vi "数据库更新.vi"(0 "设备号":string(combo)="01", 5 "数据":string[](array[string])=["123456", "ZHANG", "1", "1", "20150718", "20150719", "5", "Q14073-01", "100", "100", "100", "100", "200", "200", "200", "300", "300", "300", "300", "300", "300", "300", "300"], 11 "error in (no error)":errorcluster) -> (15 "error out":errorcluster)   [LabVIEW 2013]
panel:
  out "连接的字符串":string
  in  "数据名":string[](array[string])=["CZZ", "WC", "HG", "KSSJ", "JSSJ", "FGCS", "SBID", "Date1", "Date2", "Date3", "Date4", "Date5", "Date6", "Date7", "Date8", "Date9", "Date10"]
  # "CZZ\nWC\nHG\nKSSJ\nJSSJ\nFGCS\nSBID\nDate1\nDate2\nDate3\nDate4\nDate5\nDate6\nDate7\nDate8\nDate9\nDate10"
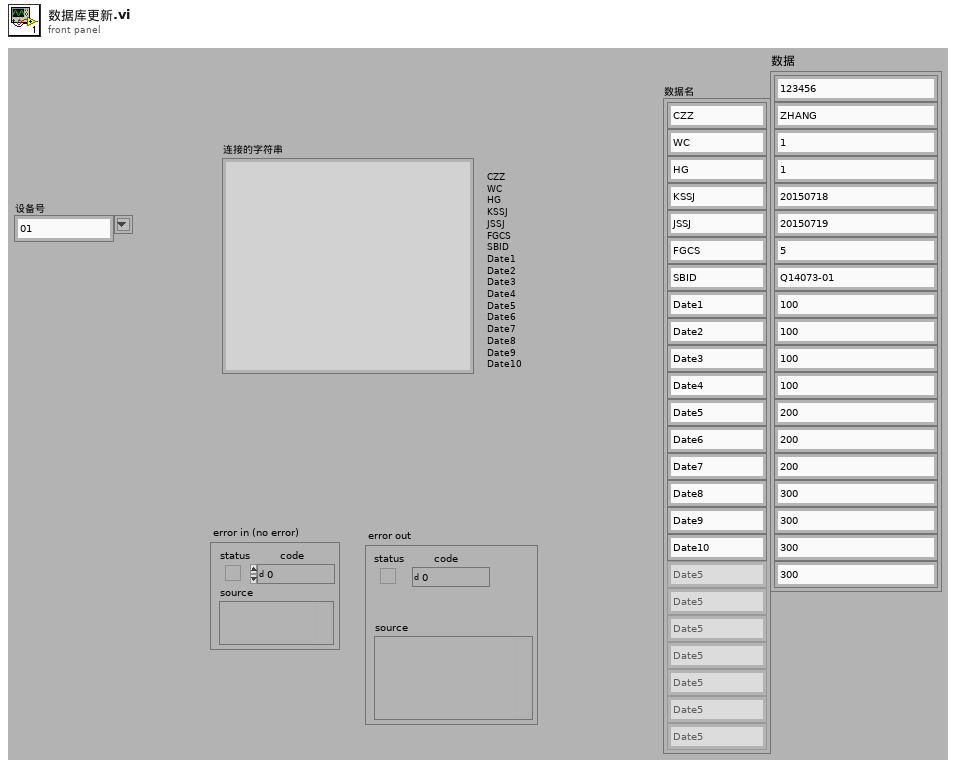
[diagram p1: front panel]
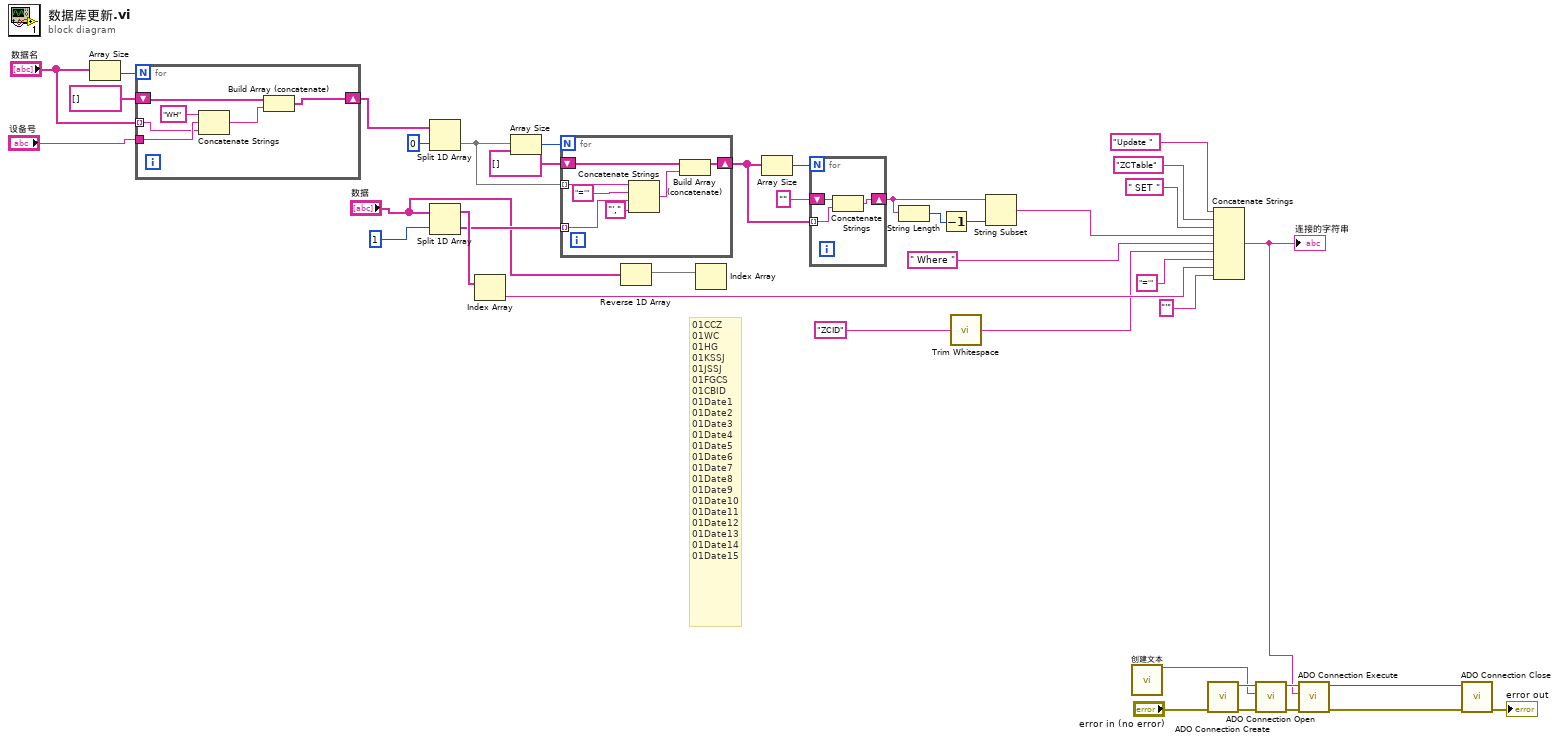
[diagram p0: block diagram]
diagram:
  # "01CCZ\n01WC\n01HG\n01KSSJ\n01JSSJ\n01FGCS\n01CBID\n01Date1\n01Date2\n01Date3\n01Date4\n01Date5\n01Date6\n01Date7\n01Date8\n01Date9\n01Date10\n01Date11\n01Date12\n01Date13\n01Date14\n01Date15"
  n1 = Array Size(array="数据名") -> (size(s)=w12:i32)
  n2 = for {
    N: w12 -> [_]
    tunnel: "数据名" -> [w42] mode=indexing
    shift-right: [w44] -> w8
    shift-left: string[] [] -> [w46]
    tunnel: "设备号" -> [w43]
    n3 = Concatenate Strings("WH" ("字符串"), w43, w42) -> (w45:string)
    n4 = Build Array (concatenate)(w46, w45) -> (w44:string[])
  }
  n5 = Split 1D Array(array=w8, index=0 ("索引")) -> (second subarray=w28:string[])  [unwired: 1 out]
  n6 = Split 1D Array(array="数据", index=1 ("索引列")) -> (first subarray=w30:string[], second subarray=w27:string[])
  n7 = Index Array(array=w30) -> (element=w15:string)  [unwired: 1 in]
  n8 = Array Size(array=w28) -> (size(s)=w29:i32)
  n9 = for {
    N: w29 -> [_]
    tunnel: w28 -> [w53] mode=indexing
    shift-right: [w50] -> w25
    shift-left: string[] [] -> [w49]
    tunnel: w27 -> [w48] mode=indexing
    n10 = Concatenate Strings(w53, "='" ("字符串"), w48, "'," ("字符串")) -> (w51:string)
    n11 = Build Array (concatenate)(w49, w51) -> (w50:string[])
  }
  n12 = Reverse 1D Array(array="数据") -> (reversed array=w7:string[])
  n13 = Index Array(array=w7) -> ()  [unwired: 1 in, 1 out]
  n14 = Array Size(array=w25) -> (size(s)=w26:i32)
  n15 = for {
    N: w26 -> [_]
    tunnel: w25 -> [w56] mode=indexing
    shift-right: [w55] -> w24
    shift-left: "" -> [w54]
    n16 = Concatenate Strings(w54, w56) -> (w55:string)
  }
  n17 = String Length(string=w24) -> (length=w5:i32)
  n18 = Decrement(x=w5) -> (x-1=w4:i32)
  n19 = call <vilib>:"Trim Whitespace.vi"("string"="ZCID" ("索引列名")) -> ("trimmed string"=w1:string)  [unwired: 1 in]
  n20 = String Subset(string=w24, length (rest)=w4) -> (substring=w3:string)  [unwired: 1 in]
  n21 = call "创建文本"() -> ("Result"=w32:string)  [unwired: 14 in, 1 out]
  n22 = call "ADO Connection Create.vi"("error in (no error)"="error in (no error)") -> ("error out"=w39:errorcluster, "ADODB._Connection Out"=w38:refnum<k7>)  [unwired: 9 out]
  n23 = Concatenate Strings("Update " ("字符串"), "ZCTable" ("数据库名"), " SET " ("字符串"), w3, " Where " ("字符串"), w1, "='" ("字符串"), w15, "'" ("字符串")) -> (w6:string)
  "连接的字符串" <- w6
  n24 = call "ADO Connection Open.vi"("error in (no error)"=w39, "ConnectionString"=w32, "ADODB._Connection In"=w38) -> ("error out"=w37:errorcluster, "ADODB._Connection Out"=w36:refnum<k7>)  [unwired: 7 out]
  n25 = call "ADO Connection Execute.vi"("error in (no error)"=w37, "CommandText"=w6, "ADODB._Connection In"=w36) -> ("error out"=w35:errorcluster, "ADODB._Connection Out"=w34:refnum<k7>)  [unwired: 7 out]
  n26 = call "ADO Connection Close.vi"("error in (no error)"=w35, "ADODB._Connection In"=w34) -> ("error out"=→"error out":errorcluster)  [unwired: 9 out]
